vi "DG - Get acquisition data.vi"(2 "error in":errorcluster, 3 "Address / Port":i16=1 min=1 max=31 step=1) -> (0 "error out":errorcluster, 1 "Data collected":dbl format="%.2f")   [LabVIEW 2014]
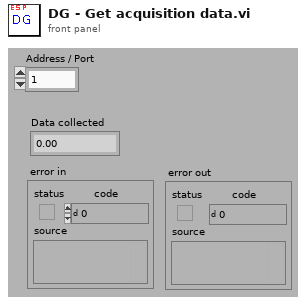
[diagram p1: front panel]
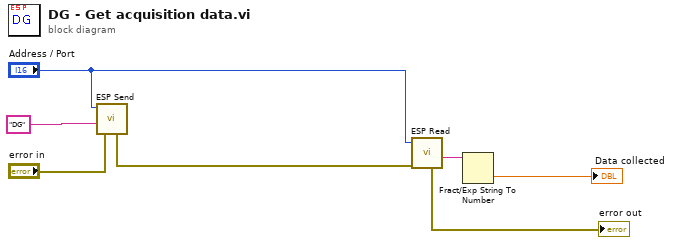
[diagram p0: block diagram]
diagram:
  n1 = call "ESP Send.vi"("Address / Port"="Address / Port", "Command String"="DG" ("Substring"), "error in"="error in") -> ("error out"=w3:errorcluster)  [unwired: 5 in]
  n2 = call "ESP Read.vi"("Address / Port"="Address / Port", "error in"=w3) -> ("error out"=→"error out":errorcluster, "Response String"=w5:string)  [unwired: 5 in]
  n3 = Fract/Exp String To Number(string=w5) -> (number=→"Data collected":dbl)  [unwired: 3 in, 1 out]
